vi "Initialize.vi"(8 "error in (no error)":errorcluster, 9 "Device":string, 10 "VISA Com Port":refnum<visa-resource-name>, 11 "NXP in":refnum<class "NXP.lvclass">) -> (0 "error out":errorcluster, 3 "NXP out":refnum<class "NXP.lvclass">)   [LabVIEW 2020, in "NXP.lvclass"]
uses:
  NXP.lvclass
  NXP.lvclass/NXP.ctl
  <vilib>/Instr/_visa.llb/VISA Configure Serial Port (Instr).vi
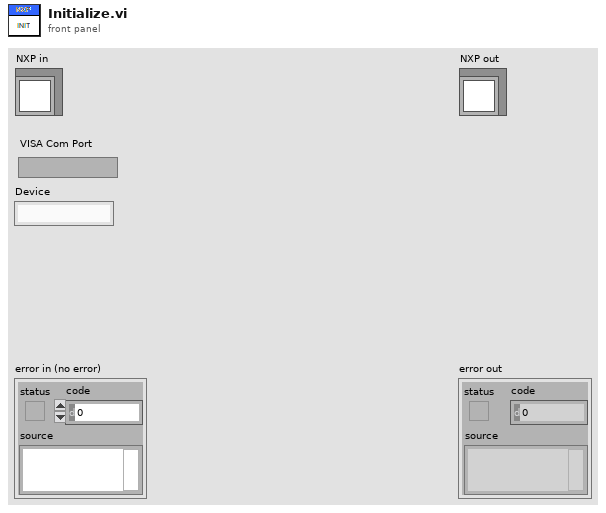
[diagram p1: front panel]
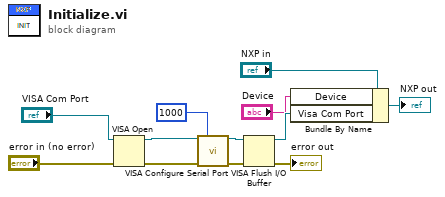
[diagram p0: block diagram]
diagram:
  n1 = VISA Open(error in (no error)="error in (no error)", VISA resource name="VISA Com Port") -> (VISA resource name=w11:refnum<visa-resource-name>, error out=w12:errorcluster)  [unwired: 3 in]
  n2 = call-poly "VISA Configure Serial Port"("VISA resource name"=w11, "timeout (10sec)"=u32 1000, "error in (no error)"=w12) -> ("VISA resource name out"=w10:refnum<visa-resource-name>, "error out"=w8:errorcluster)  [unwired: 11 in]
  n3 = VISA Flush I/O Buffer(VISA resource name=w10, error in (no error)=w8) -> (VISA resource name out=w9:refnum<visa-resource-name>, error out=→"error out":errorcluster)  [unwired: 1 in]
  n4 = Bundle By Name(cluster="NXP in", "Device"="Device", "Visa Com Port"=w9) -> (→"NXP out":refnum<class "NXP.lvclass">)
